vi "SerialClose.vi"(8 "error in (no error)":errorcluster caption="错误输入（无错误）", 11 "serial 输入":refnum<class "serial.lvclass">) -> (0 "error out":errorcluster caption="错误输出", 3 "serial 输出":refnum<class "serial.lvclass">)   [LabVIEW 2019, in "serial.lvclass"]
uses:
  serial.lvclass
  serial.lvclass/serial.ctl
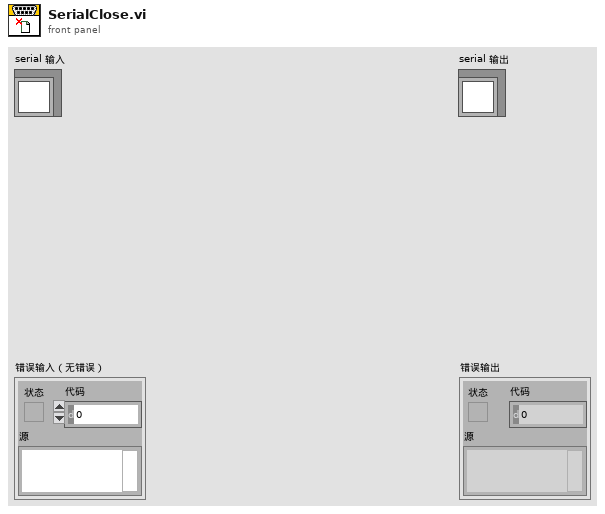
[diagram p1: front panel]
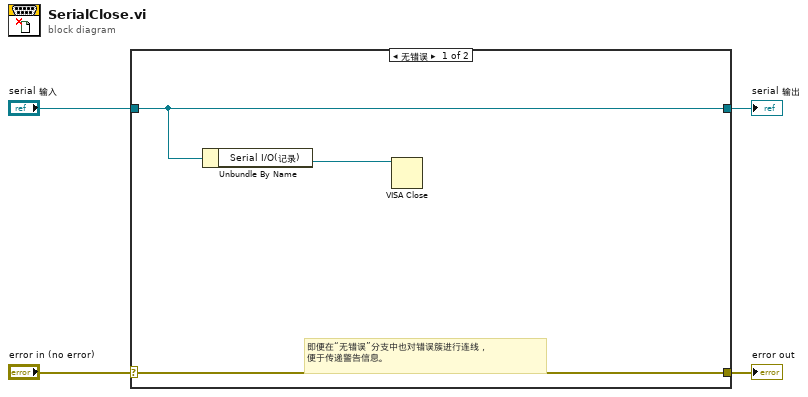
[diagram p0: block diagram]
diagram:
  n1 = case shown="无错误" "error in (no error)" {
    selector: "error in (no error)" -> [w7 w9]
    tunnel: [w7 w9] -> w3
    tunnel: [w6 w8] -> w1
    tunnel: "serial 输入" -> [w6 w8]
    frame No Error {
      # "即便在“无错误”分支中也对错误簇进行连线，\n便于传递警告信息。"
      n2 = Unbundle By Name(w6) -> ("Serial I/O(记录)"=w5:refnum<visa-resource-name>)
      n3 = VISA Close(VISA resource name=w5) -> ()  [unwired: 1 in, 1 out]
    }
    frame Error {
    }
  }
  "error out" <- w3
  "serial 输出" <- w1
